vi "Read Directors.vi"(8 "error in (no error)":errorcluster, 11 "InteractionProcessor in":refnum<class "InteractionProcessor.lvclass">) -> (0 "error out":errorcluster, 2 "Directors":refnum<class "CommandDirector.lvclass">[](array[class]), 3 "InteractionProcessor out":refnum<class "InteractionProcessor.lvclass">)   [LabVIEW 2023, in "HAF.lvlib" / "InteractionProcessor.lvclass"]
doc: "Returns the current collection of CommandDirectors."
uses:
  InteractionProcessor.lvclass
  CommandDirector/CommandDirector.lvclass
  InteractionProcessor.lvclass/InteractionProcessor.ctl
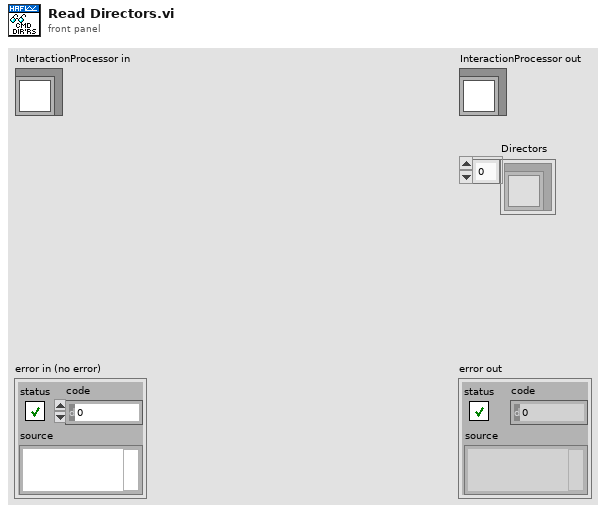
[diagram p1: front panel]
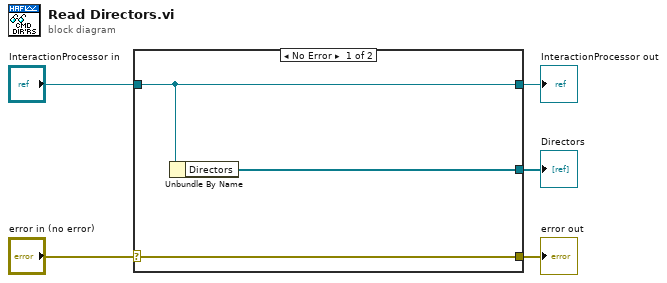
[diagram p0: block diagram]
diagram:
  n1 = case shown="No Error" "error in (no error)" {
    selector: "error in (no error)" -> [w8 w9]
    tunnel: [w8 w9] -> w4
    tunnel: [w7 w10] -> w2
    tunnel: "InteractionProcessor in" -> [w7 w10]
    tunnel: [w6 _] -> w1
    frame No Error {
      n2 = Unbundle By Name(w7) -> ("Directors"=w6:refnum<class "CommandDirector.lvclass">[])
    }
    frame Error {
    }
  }
  "error out" <- w4
  "InteractionProcessor out" <- w2
  "Directors" <- w1
